vi "ClusterExperiment.vi"() -> ()   [LabVIEW 2014]
panel:
  out "Numeric":dbl
  in  "stop":bool
  out "Boolean":bool
  out "Cluster 3":cluster{"Boolean":bool, "Numeric":dbl}
  out "Cluster 2":T1 {"Slide" scale=0.0..10.0}
  in  "Cluster":T1 {"Slide" scale=0.0..10.0}
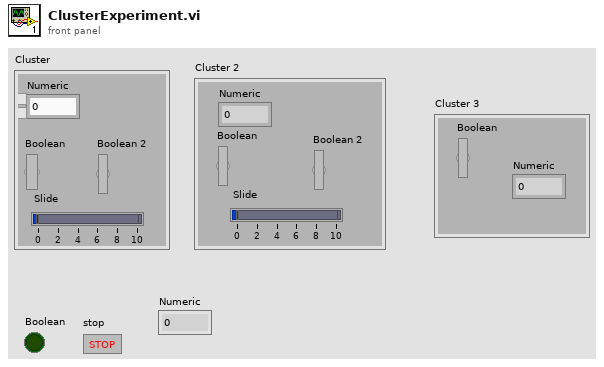
[diagram p1: front panel]
types:
  T1 = cluster{"Numeric":dbl, "Boolean":bool, "Boolean 2":bool, "Slide":dbl}
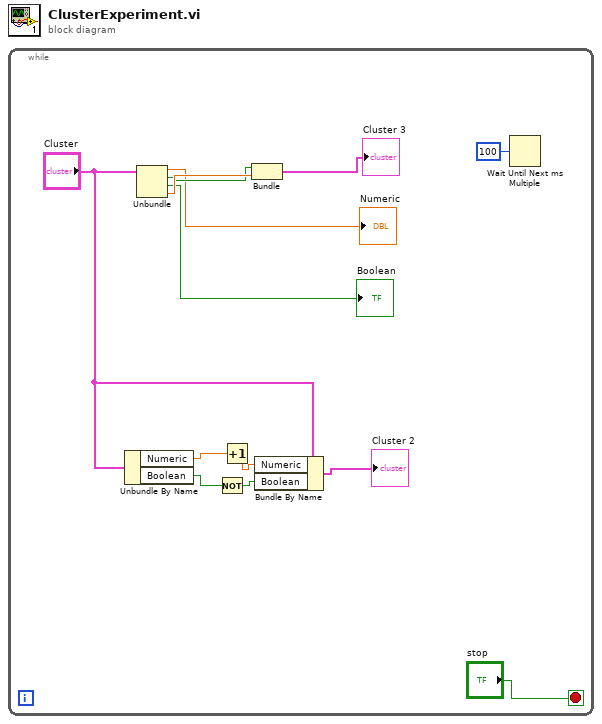
[diagram p0: block diagram]
diagram:
  n1 = while {
    stop <- "stop" stop-if-true
    n2 = Unbundle By Name("Cluster") -> ("Numeric"=w5:dbl, "Boolean"=w4:bool)
    n3 = Unbundle("Cluster") -> ("Numeric"=→"Numeric":dbl, "Boolean"=w11:bool, "Boolean 2"=→"Boolean":bool, "Slide"=w12:dbl)
    n4 = Not(x=w4) -> (.not. x?=w3:bool)
    n5 = Increment(x=w5) -> (x+1=w2:dbl)
    n6 = Bundle("Boolean"=w11, "Slide"=w12) -> (→"Cluster 3":cluster{"Boolean":bool, "Slide":dbl})  [unwired: 1 in]
    n7 = Bundle By Name(cluster="Cluster", "Numeric"=w2, "Boolean"=w3) -> (→"Cluster 2":T1)
    n8 = Wait Until Next ms Multiple(millisecond multiple=u32 100) -> ()  [unwired: 1 out]
  }
